vi "Test CSRF.vi"() -> ()   [LabVIEW 2020]
uses:
  lv-http-server/HTTP Server/Trace Log.ctl
  lv-http-server/HTTP Server/Trace Item.ctl
  lv-http-server/HTTP Server/Processing Step.ctl
  lv-http-util/HTTP Utils/Method.ctl
  TestCSRFController/TestCSRFController.lvclass
  C:/dev/lv20CE/relink/lv-http-server/HTTP Server/Handler/Handler.lvclass
  lv-http-server/HTTP Server/Server/Add Connection Handler.vi
  lv-http-server/HTTP Server/Server/Add Request Handler.vi
  lv-http-server/HTTP Server/Server/Add Route Handler.vi
  lv-http-server/HTTP Server/Server/Add Controller Handler.vi
  lv-http-server/HTTP Server/Server/Add Controller.vi
  lv-http-server/HTTP Server/Server/Add Response Handler.vi
  lv-http-server/HTTP Server/Server/Add Complete Handler.vi
  lv-http-server/HTTP Server/Server/Add Exception Handler.vi
  lv-http-server/HTTP Server/Connection Handler/Connection Handler.lvclass
  lv-http-server/HTTP Server/Request Handler/Request Handler.lvclass
  lv-http-server/HTTP Server/Route Handler/Route Handler.lvclass
  lv-http-server/HTTP Server/Controller Handler/Controller Handler.lvclass
  lv-http-server/HTTP Server/Controller/Controller.lvclass
  lv-http-server/HTTP Server/Response Handler/Response Handler.lvclass
  lv-http-server/HTTP Server/Complete Handler/Complete Handler.lvclass
  lv-http-server/HTTP Server/Exception Handler/Exception Handler.lvclass
  lv-http-server/HTTP Server/Server/Server.lvclass
  lv-http-server/HTTP Server/Handler/Handler.lvclass
  lv-http-server/HTTP Server/RequestTraceLog/RequestTraceLog.lvclass
  lv-http-server/HTTP Server/Session/Session.lvclass
  lv-http-server/HTTP Server/HTTP Server.lvlib
  lv-http-util/HTTP Utils/HTTP Utils.lvlib
panel:
  out "error out":errorcluster
  in  "Debug":bool=TRUE
  in  "Refresh Traces":bool
  out "Traces":T1[](array[typedef]) {"Sending" format="%_6f"; "Expires" format="%<%X %x>T"; "Created" format="%<%X %x>T"; "Waiting" format="%_6f"; "Parsing" format="%_6f"; "Processing" format="%_6f"; "Items"."Time" format="%.6f"; "Items"."Duration" format="%.6f"}
  in  "Port":u16=36987
  # "Request"
  # "Response"
  # "Session"
  # "Auth"
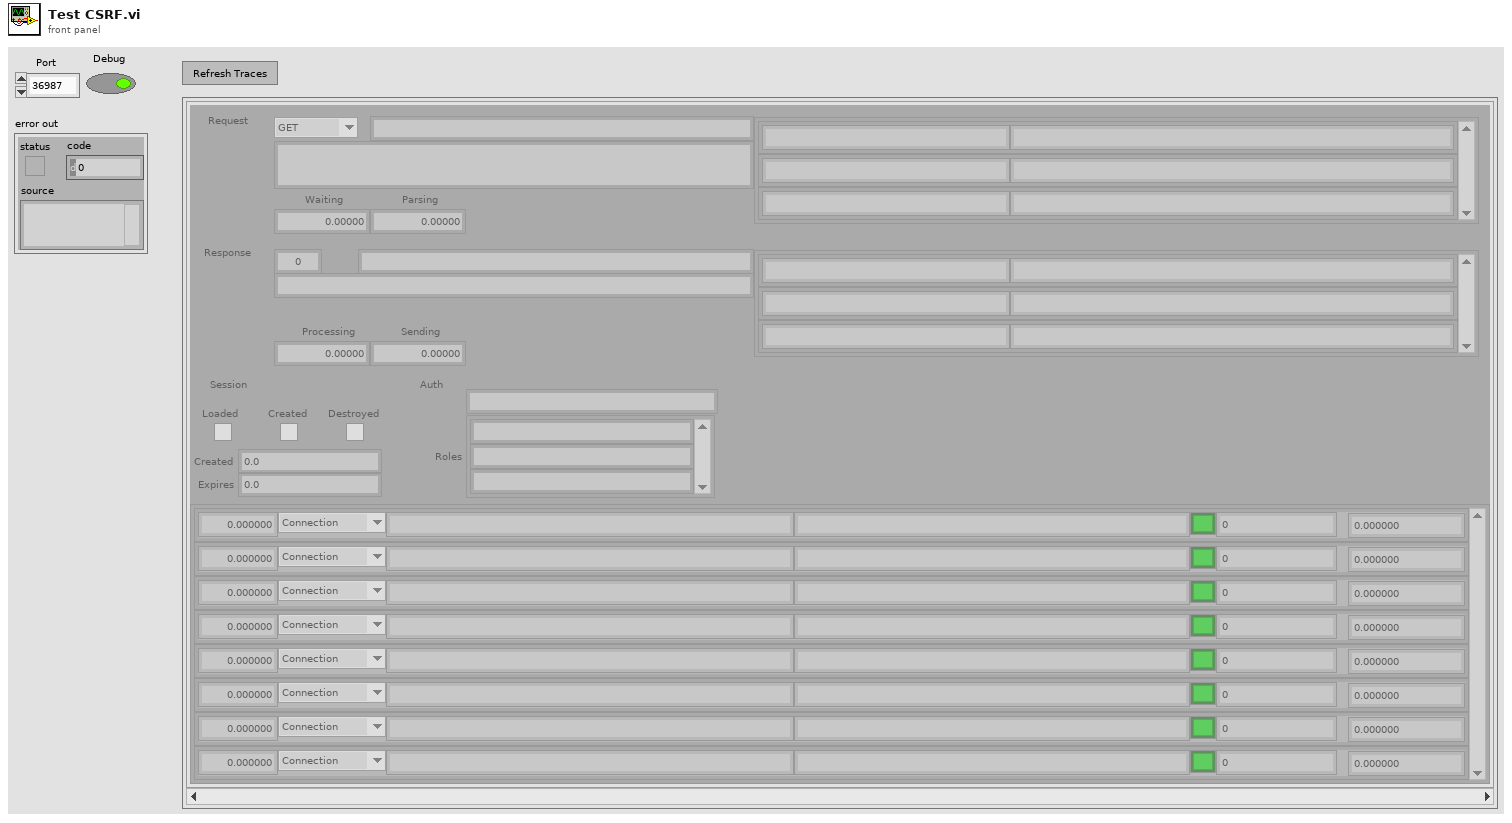
[diagram p1: front panel]
types:
  T1 = typedef "HTTP Server.lvlib/Trace Log.ctl" = cluster{"Items":T2[], "Client":string, "Target":string, "Response Type":string, "Processing":dbl, "Status":u16, "Method":T4, "Content Type":string, "Request Headers":cluster{"Name":string, "Value":string}[], "Parsing":dbl, "Waiting":dbl, "Identity":string, "Loaded":bool, "Created":bool, "Destroyed":bool, "Response Headers":cluster{"Name":string, "Value":string}[], "Created":dbl, "Expires":dbl, "Roles":string[], "Sending":dbl}
  T2 = typedef "HTTP Server.lvlib/Trace Item.ctl" = cluster{"Duration":dbl, "Step":T3, "Class":string, "Info":string, "Status":bool, "Code":i32, "Time":dbl}
  T3 = typedef "HTTP Server.lvlib/Processing Step.ctl" = enum16{"Connection", "Request", "Routing", "Controller Init", "Controller", "Response", "Complete", "Exception"}
  T4 = typedef "HTTP Utils.lvlib/Method.ctl" = enum16{"GET", "HEAD", "POST", "PUT", "DELETE", "CONNECT", "OPTIONS", "TRACE", "PATCH"}
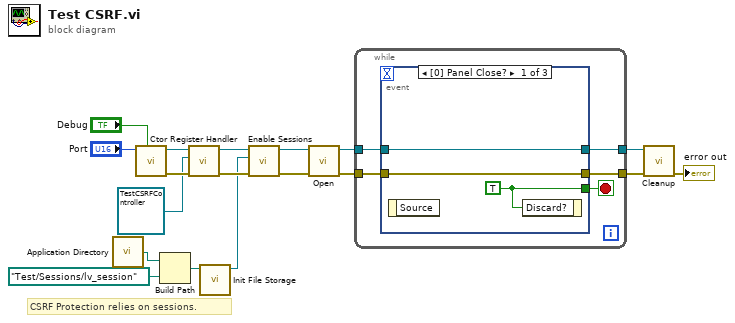
[diagram p0: block diagram]
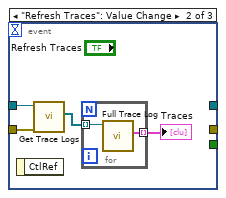
[diagram p2: hidden frame]
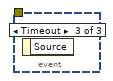
[diagram p3: hidden frame]
diagram:
  # "CSRF Protection relies on sessions."
  n1 = call <vilib>:"Application Directory.vi"() -> ("Application Directory"=w8:path)
  n2 = call "Ctor.vi"("Debug (F)"="Debug", "HTTP Port (80)"="Port") -> ("error out"=w11:errorcluster, "Server out"=w12:refnum<class "Server.lvclass">)  [unwired: 8 in]
  n3 = Build Path(base path=w8, name or relative path=path "Test/Sessions/lv_session") -> (appended path=w6:path)
  n4 = call "Register Handler.vi"("error in (no error)"=w11, "Handler"=refnum<class "TestCSRFController.lvclass"> refnum ("TestCSRFController.lvclass"), "Server in"=w12) -> ("error out"=w4:errorcluster, "Server out"=w5:refnum<class "Server.lvclass">)  [unwired: 7 in]
  n5 = call "Init File Storage.vi"("Session Storage Folder"=w6) -> ("Session out"=w1:refnum<class "Session.lvclass">)  [unwired: 9 in, 1 out]
  n6 = call "Enable Sessions.vi"("error in (no error)"=w4, "Session Implementation"=w1, "Server in"=w5) -> ("error out"=w3:errorcluster, "Server out"=w2:refnum<class "Server.lvclass">)  [unwired: 7 in]
  n7 = call "Open.vi"("error in (no error)"=w3, "Server in"=w2) -> ("error out"=w16:errorcluster, "Server out"=w17:refnum<class "Server.lvclass">)  [unwired: 8 in]
  n8 = while {
    tunnel: w17 -> [w21]
    tunnel: w16 -> [w22]
    tunnel: [w20] -> w15
    tunnel: [w19] -> w14
    stop <- w23 stop-if-true
    n9 = event shown="[0] Panel Close?" {
      selector: _ -> [_ _ _]
      dyn-events: _ -> [_ _ _]
      timeout: _ -> [_ _ _]
      tunnel: [w24 _ _] -> w23
      tunnel: w22 -> [w25 w29 _]
      tunnel: w21 -> [w26 w30 _]
      tunnel: [w26 _ _] -> w20
      tunnel: [w25 _ _] -> w19
      event Panel Close? {
        w24 = TRUE ("Discard?")
        n10 = event-data() -> ()  [unwired: 1 in, 1 out]
        n11 = event-data("Discard?"=w24) -> ()  [unwired: 1 in, 1 out]
      }
      event "Refresh Traces": Value Change {
        n12 = event-data() -> ()  [unwired: 1 in, 1 out]
        n13 = call "Get Trace Logs.vi"("error in (no error)"=w29, "Server in"=w30) -> ("Trace Logs"=w28:refnum<class "RequestTraceLog.lvclass">[])  [unwired: 7 in, 2 out]
        n14 = for {
          tunnel: w28 -> [w32] mode=indexing
          tunnel: [w31] -> w27 mode=indexing
          n15 = call "Full Trace Log.vi"("RequestTraceLog in"=w32) -> ("Trace Log"=w31:T1)  [unwired: 8 in, 2 out]
        }
        "Traces" <- w27
      }
      event Timeout {
        n16 = event-data() -> ()  [unwired: 1 in, 1 out]
      }
    }
  }
  n17 = call "Cleanup.vi"("error in (no error)"=w14, "Server in"=w15) -> ("error out"=→"error out":errorcluster)  [unwired: 9 in]
